vi "write_file_test.vi"() -> ()   [LabVIEW 2016]
uses:
  <vilib>/Utility/file.llb/Write Delimited Spreadsheet (DBL).vi
  <vilib>/LabVIEW Interface for Arduino/LabVIEW Interface for Arduino.lvlib
panel:
  in  "transpose? (no:F) 2":bool
  in  "append to file? (new file:F) 2":bool
  in  "transpose? (no:F)":bool
  in  "append to file? (new file:F)":bool
  out "Voltage":dbl(knob) scale=0.0..5.0
  out "Numeric":i32
  in  "stop":bool
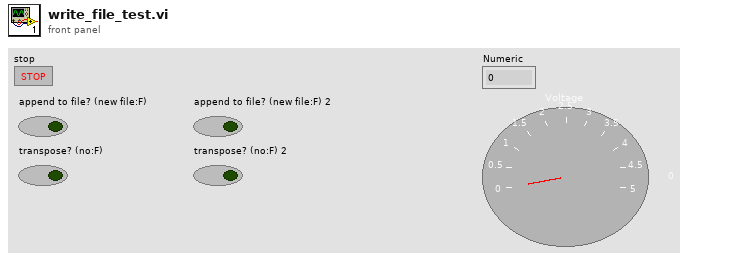
[diagram p1: front panel]
types:
  T1 = typedef "LabVIEW Interface for Arduino.lvlib/Arduino Resource.ctl" = cluster{"VISA resource":refnum<visa-resource-name>, "Board Type":T2, "Connection Type":enum8{"USB / Serial"}, "Bytes Per Packet (15)":u8}
  T2 = typedef "LabVIEW Interface for Arduino.lvlib/Board Type.ctl" = enum16{"Uno", "Dimuelanove w/Atmega 328", "Mega 2560"}
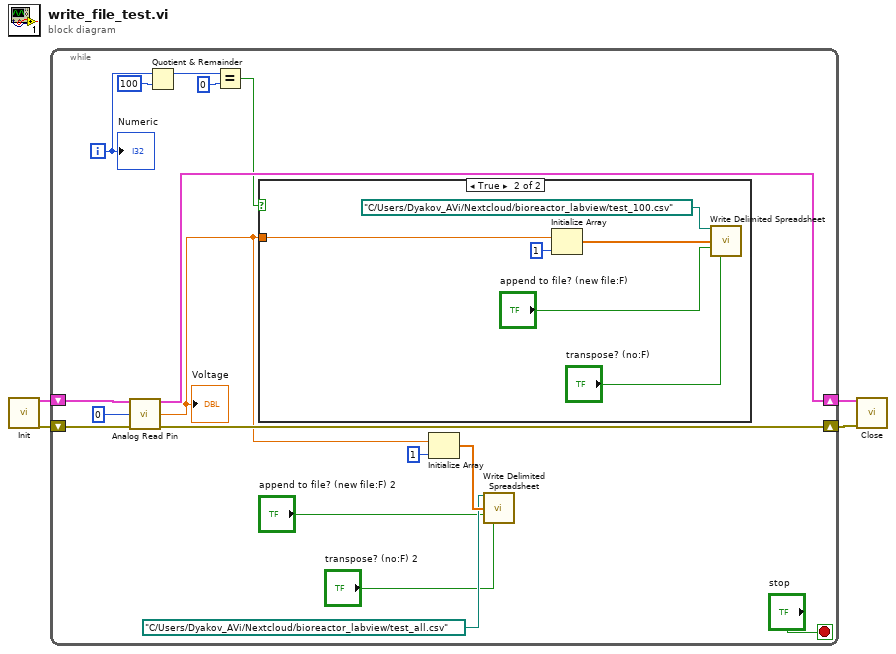
[diagram p0: block diagram]
diagram:
  n1 = call <vilib>:"Init.vi"() -> ("Arduino Resource"=w4:T1, "error out"=w2:errorcluster)  [unwired: 18 in]
  n2 = while {
    shift-right: [w19] -> w3
    shift-left: w4 -> [w20]
    shift-right: [w17] -> w1
    shift-left: w2 -> [w18]
    i -> [w15]
    stop <- "stop" stop-if-true
    n3 = call <vilib>:"Analog Read Pin.vi"("Arduino Resource"=w20, "Analog Input Pin (0)"=u8 0, "error in"=w18) -> ("Arduino Resource"=w19:T1, "Voltage"=w6:dbl, "error out"=w17:errorcluster)  [unwired: 10 in]
    "Voltage" <- w6
    n4 = Quotient & Remainder(x=w15, y=100) -> (x-y*floor(x/y)=w13:i32)  [unwired: 1 out]
    n5 = Equal?(x=w13, y=0) -> (x = y?=w11:bool)
    n6 = case shown="True" w11 {
      tunnel: w6 -> [_ w27]
      frame False {
      }
      frame True {
        n7 = Initialize Array(w27, 1 ("dimension size")) -> (w26:dbl[])
        n8 = call-poly <vilib>:"Write Delimited Spreadsheet.vi"("file path (dialog if empty)"=path "C:/Users/Dyakov_AVi/Nextcloud/bioreactor_labview/test_100.csv", "1D data"=w26, "append to file? (new file:F)"="append to file? (new file:F)", "transpose? (no:F)"="transpose? (no:F)") -> ()  [unwired: 10 in, 2 out]
      }
    }
    n9 = Initialize Array(w6, 1 ("dimension size")) -> (w10:dbl[])
    n10 = call-poly <vilib>:"Write Delimited Spreadsheet.vi"("file path (dialog if empty)"=path "C:/Users/Dyakov_AVi/Nextcloud/bioreactor_labview/test_all.csv", "1D data"=w10, "append to file? (new file:F)"="append to file? (new file:F) 2", "transpose? (no:F)"="transpose? (no:F) 2") -> ()  [unwired: 10 in, 2 out]
    "Numeric" <- w15
  }
  n11 = call <vilib>:"Close.vi"("Arduino Resource"=w3, "error in"=w1) -> ()  [unwired: 13 in, 1 out]
